vi "OAXML_Data Logger Configuration.vi"(8 "DAQ Config in":T1 {"pregain" format="%.2f"; "IEPE" items=["On", "Off", "None"]; "coupling" items=["DC", "AC"]; "engineering units" items=["custom..."=0, "V"=1, "A"=21, "C"=30, "pC"=31, "s"=32, "-"=29, "Pa"=2, "N"=20, "g"=3, "m/s^2"=4, "m/s"=5, "m"=6, "mm/s"=12, "mm"=13, "micron/s"=14, "micron"=15, "in/s^2"=7, "in/s"=8, "in"=9, "mil/s"=10, "mil"=11, "rad/s^2"=16, "rad/s"=17, "rad"=18, "deg/s^2"=26, "deg/s"=27, "deg"=28, "RPM"=22, "cycle/s^2"=23, "Hz"=24, "cycle"=25, "strain"=19]; "sensor sensitivity (mV/EU)" format="%.2f"; "dB reference" format="%.1e"}, 11 "Param in":T3={"tachometer channel"="", "sample rate [samples/s]"=10000.0, "Max Value"=5.0, "Min Value"=-5.0, "Path"=path ""} {"Min Value" format="%0.2f"; "Max Value" format="%0.2f"}) -> (0 "DAQ Config out":T1 {"pregain" format="%.2f"; "IEPE" items=["On", "Off", "None"]; "coupling" items=["DC", "AC"]; "engineering units" items=["custom..."=0, "V"=1, "A"=21, "C"=30, "pC"=31, "s"=32, "-"=29, "Pa"=2, "N"=20, "g"=3, "m/s^2"=4, "m/s"=5, "m"=6, "mm/s"=12, "mm"=13, "micron/s"=14, "micron"=15, "in/s^2"=7, "in/s"=8, "in"=9, "mil/s"=10, "mil"=11, "rad/s^2"=16, "rad/s"=17, "rad"=18, "deg/s^2"=26, "deg/s"=27, "deg"=28, "RPM"=22, "cycle/s^2"=23, "Hz"=24, "cycle"=25, "strain"=19]; "sensor sensitivity (mV/EU)" format="%.2f"; "dB reference" format="%.1e"}, 1 "result":u16(ring) items=["OK", "Cancel"], 3 "Param out":T3={"tachometer channel"="", "sample rate [samples/s]"=10000.0, "Max Value"=5.0, "Min Value"=-5.0, "Path"=path ""} {"Min Value" format="%0.2f"; "Max Value" format="%0.2f"})   [LabVIEW 2017]
uses:
  <vilib>/addons/Sound and Vibration/Order Analysis/Example Support/sub VIs/OAXML_DSA DAQ Config.ctl
  <vilib>/addons/_NISVFA/_Shared subVIs/Controls/svc_Engineering Units Text Ring.ctl
panel:
  in  "Cancel":bool
  in  "OK":bool
  in  "Path":path
  in  "tachometer channel":tag
  in  "sample rate [samples/s]":dbl=10000.0 min=1.0 step=1.0
  in  "Min Value":dbl=-5.0 format="%0.2f"
  in  "Max Value":dbl=5.0 format="%0.2f"
  in  "DAQ Config":T1 {"pregain" format="%.2f"; "IEPE" items=["On", "Off", "None"]; "coupling" items=["DC", "AC"]; "engineering units" items=["custom..."=0, "V"=1, "A"=21, "C"=30, "pC"=31, "s"=32, "-"=29, "Pa"=2, "N"=20, "g"=3, "m/s^2"=4, "m/s"=5, "m"=6, "mm/s"=12, "mm"=13, "micron/s"=14, "micron"=15, "in/s^2"=7, "in/s"=8, "in"=9, "mil/s"=10, "mil"=11, "rad/s^2"=16, "rad/s"=17, "rad"=18, "deg/s^2"=26, "deg/s"=27, "deg"=28, "RPM"=22, "cycle/s^2"=23, "Hz"=24, "cycle"=25, "strain"=19]; "sensor sensitivity (mV/EU)" format="%.2f"; "dB reference" format="%.1e"}
  # "DAQ Configuration"
  # "Folder for saving data"
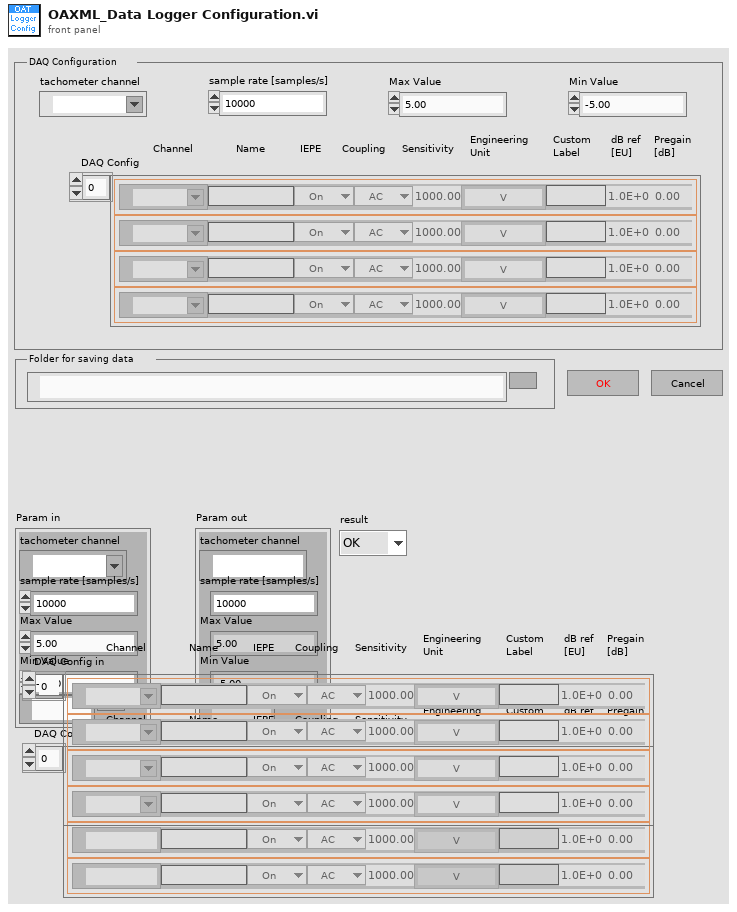
[diagram p1: front panel]
types:
  T1 = typedef "OAXML_DSA DAQ Config.ctl" = cluster{"name":string, "channel":tag, "coupling":u16, "dB reference":sgl, "sensor sensitivity (mV/EU)":dbl, "engineering units":T2, "IEPE":u16, "custom label":string, "pregain":sgl}[]
  T2 = typedef "svc_Engineering Units Text Ring.ctl" = u16
  T3 = cluster{"tachometer channel":tag, "sample rate [samples/s]":dbl, "Max Value":dbl, "Min Value":dbl, "Path":path}
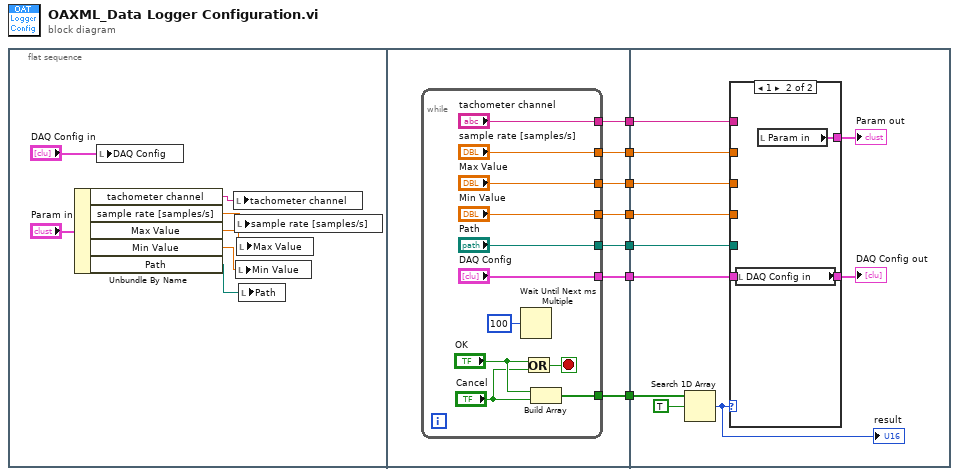
[diagram p0: block diagram]
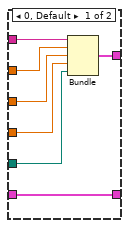
[diagram p2: hidden frame]
diagram:
  n1 = flat-sequence {
    tunnel: [w21] -> w7
    tunnel: [w20] -> w6
    tunnel: [w19] -> w5
    tunnel: [w18] -> w4
    tunnel: [w17] -> w3
    tunnel: [w16] -> w2
    tunnel: [w15] -> w1
    tunnel: w7 -> [w43]
    tunnel: w6 -> [w42]
    tunnel: w5 -> [w41]
    tunnel: w4 -> [w40]
    tunnel: w3 -> [w39]
    tunnel: w2 -> [w38]
    tunnel: w1 -> [w37]
    frame #0 {
      n2 = Unbundle By Name("Param in") -> ("tachometer channel"=w12:tag, "sample rate [samples/s]"=w11:dbl, "Max Value"=w10:dbl, "Min Value"=w9:dbl, "Path"=w8:path)
      n3 = local write "DAQ Config"("DAQ Config in") -> ()
      n4 = local write "tachometer channel"(w12) -> ()
      n5 = local write "sample rate [samples/s]"(w11) -> ()
      n6 = local write "Min Value"(w9) -> ()
      n7 = local write "Max Value"(w10) -> ()
      n8 = local write "Path"(w8) -> ()
    }
    frame #1 {
      n9 = while {
        tunnel: ["tachometer channel"] -> w21
        tunnel: ["sample rate [samples/s]"] -> w20
        tunnel: ["Max Value"] -> w19
        tunnel: ["Min Value"] -> w18
        tunnel: ["Path"] -> w17
        tunnel: ["DAQ Config"] -> w16
        tunnel: [w22] -> w15
        stop <- w25 stop-if-true
        n10 = Wait Until Next ms Multiple(millisecond multiple=u32 100) -> ()  [unwired: 1 out]
        n11 = Or(x="OK", y="Cancel") -> (x .or. y?=w25:bool)
        n12 = Build Array("OK", "Cancel") -> (w22:bool[])
      }
    }
    frame #2 {
      n13 = Search 1D Array(1D array=w37, element=TRUE ("Cancel")) -> (index of element=w33:i32)  [unwired: 1 in]
      "result" <- w33
      n14 = case shown="1" w33 {
        tunnel: w43 -> [w50 _]
        tunnel: w42 -> [w49 _]
        tunnel: w41 -> [w48 _]
        tunnel: w40 -> [w47 _]
        tunnel: w39 -> [w46 _]
        tunnel: w38 -> [w44 _]
        tunnel: [w45 w51] -> w34
        tunnel: [w44 w52] -> w35
        frame 0, Default {
          n15 = Bundle("tachometer channel"=w50, "sample rate [samples/s]"=w49, "Max Value"=w48, "Min Value"=w47, "Path"=w46) -> (w45:T3)  [unwired: 1 in]
        }
        frame 1 {
          n16 = local read "DAQ Config in"() -> (w52:T1)
          n17 = local read "Param in"() -> (w51:T3)
        }
      }
      "Param out" <- w34
      "DAQ Config out" <- w35
    }
  }
